vi "LCM_logger.vi"   [LabVIEW 2015]
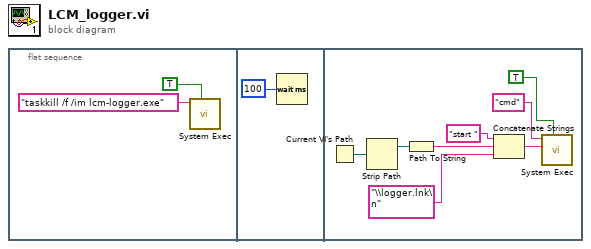
[diagram p0: block diagram]
diagram:
  n1 = flat-sequence {
    frame #0 {
      n2 = call <vilib>:"System Exec.vi"("wait until completion? (T)"=TRUE, "command line"="taskkill /f /im lcm-logger.exe") -> ()  [unwired: 6 in, 4 out]
    }
    frame #1 {
      n3 = Wait (ms)(milliseconds to wait=u32 100 ("millisecond timer value")) -> ()  [unwired: 1 out]
    }
    frame #2 {
      n4 = Current VI's Path() -> (path=w4:path)
      n5 = Strip Path(path=w4) -> (stripped path=w9:path)  [unwired: 1 out]
      n6 = Path To String(path=w9) -> (string=w8:string)
      n7 = Concatenate Strings("start " ("string"), w8, "\\logger.lnk\n" ("string")) -> (w6:string)
      n8 = call <vilib>:"System Exec.vi"("wait until completion? (T)"=TRUE, "standard input"=w6, "command line"="cmd") -> ()  [unwired: 5 in, 4 out]
    }
  }
